vi "CleanFieldsWithAutoKey.vi"(9 "AutoKey":string, 10 "RequestedFields":string[](array[string]), 11 "FieldNames":string[](array[string])) -> (2 "RequestedFields_Clean":string[](array[string]), 3 "FieldNames_Clean":string[](array[string]))   [LabVIEW 2020, in "ORM_DBC_Kdb.lvlib" / "DBC.lvclass"]
uses:
  DBC.lvclass
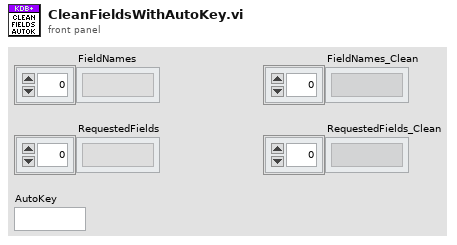
[diagram p1: front panel]
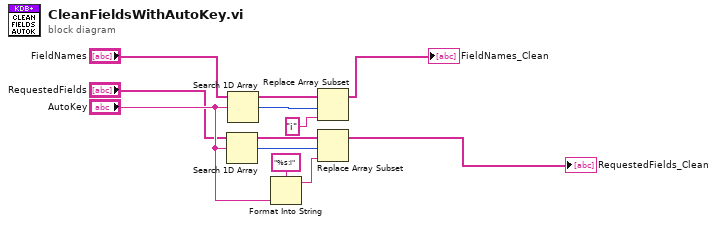
[diagram p0: block diagram]
diagram:
  n1 = Search 1D Array(1D array="RequestedFields", element="AutoKey") -> (index of element=w4:i32)  [unwired: 1 in]
  n2 = Search 1D Array(1D array="FieldNames", element="AutoKey") -> (index of element=w2:i32)  [unwired: 1 in]
  n3 = Format Into String(format string="%s:i", "AutoKey") -> (resulting string=w6:string)  [unwired: 2 in, 1 out]
  n4 = Replace Array Subset(array="FieldNames", new element="i", index=w2) -> (→"FieldNames_Clean":string[])
  n5 = Replace Array Subset(array="RequestedFields", new element=w6, index=w4) -> (→"RequestedFields_Clean":string[])
